vi "RT Main.vi"() -> ()   [LabVIEW 2021]
doc: "This example monitors the myRIO onboard button and increments or decrements the number below based on the Direction control."
uses:
  <vilib>/myRIO/Express VI/Onboard Devices/LED/LED Express VI.xnode
  <vilib>/myRIO/Instrument Drivers/Onboard IO/DIO/vis/Write.vi
  <vilib>/myRIO/Instrument Drivers/Onboard IO/DIO/DIO.lvlib
  <vilib>/myRIO/Common/Instrument Driver Framework/myRIO v1.0/DIO/typedefs/DIO Channels Enum.ctl
  <vilib>/myRIO/Common/Instrument Driver Framework/myRIO v1.0/DIO/typedefs/DIO Channels List.ctl
  <vilib>/myRIO/Common/Instrument Driver Framework/Utilities/typedefs/Generic FPGA Reference.ctl
  <vilib>/myRIO/Common/Instrument Driver Framework/Utilities/typedefs/myRIO v1.0 Reference.ctl
  <vilib>/myRIO/Common/Instrument Driver Framework/Utilities/typedefs/Hardware Version Enum.ctl
  <vilib>/myRIO/Common/Instrument Driver Framework/Utilities/typedefs/myRIO Generic Hardware Reference.ctl
  <vilib>/myRIO/Instrument Drivers/Onboard IO/DIO/typedefs/DIO Reference.ctl
  <vilib>/myRIO/Instrument Drivers/Onboard IO/DIO/vis/myRIO DIO Open.xnode
  <vilib>/myRIO/Common/Instrument Driver Framework/Utilities/vis/Is FPGA Ref Available.vi
  <vilib>/myRIO/Common/Instrument Driver Framework/myRIO v1.0/DIO/vis/myRIO v1.1 Open DIO.vi
  <vilib>/userdefined/High Color/nirio_resource_hc.ctl
panel:
  out "Axis Info":cluster{"X axis":i32, "Y axis":i32}[](graph)
  out "Pov Direction":picture
  out "Button 4":bool
  out "Button 3":bool
  out "Button 2":bool
  out "Button 1":bool
  in  "Device Index":i8
  out "error out":errorcluster
  in  "Stop":bool
  # "Overview: This VI demonstrates how to monitor the activity of the joystick connected to the myRIO.\nInstructions:\n1.\tIn the Project Explorer window, verify the IP address of the myRIO target. If it is incorrect, \nupdate the IP address.\n2. Connect a joystick to the myRIO through the USB port.\n3. Run the VI.\n4.\tPush the buttons and axes on the joystick and observe the indicators of the VI."
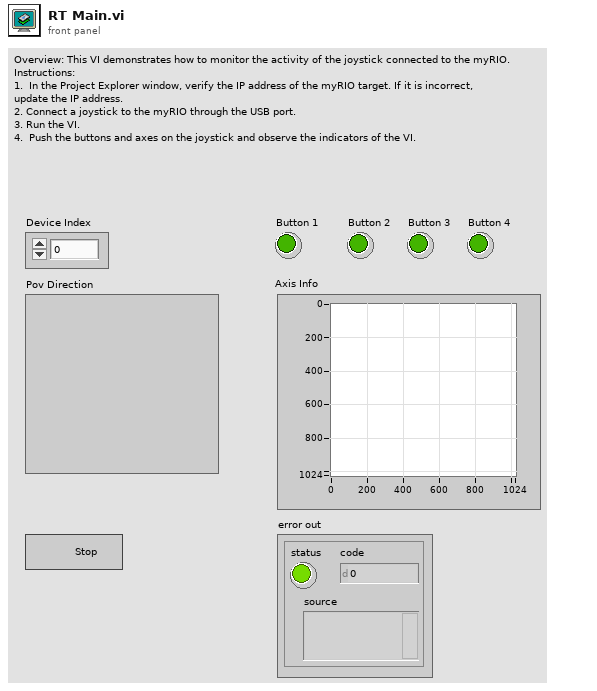
[diagram p1: front panel]
types:
  T1 = typedef "DIO.lvlib/DIO Reference.ctl" = cluster{"myRIO Reference":T2, "DIO Channels List":T6}
  T2 = typedef "myRIO Generic Hardware Reference.ctl" = cluster{"myRIO Model":T3, "myRIO Hardware Reference":T4}
  T3 = typedef "Hardware Version Enum.ctl" = enum16{"Unknown", "myRIO-1900", "myRIO-1950", "roboRIO", "NI ELVIS RIO CM", "ELVIS III"}
  T4 = typedef "myRIO v1.0 Reference.ctl" = cluster{"Generic FPGA Reference":T5, "Allow multiple opens":bool}
  T5 = typedef "Generic FPGA Reference.ctl" = refnum<k20>
  T6 = typedef "DIO Channels List.ctl" = T7[]
  T7 = typedef "DIO Channels Enum.ctl" = enum16{"Not Connected", "C/DIO0", "C/DIO1", "C/DIO2", "C/DIO3", "C/DIO4", "C/DIO5", "C/DIO6", "C/DIO7", "A/DIO0", "A/DIO1", "A/DIO2", "A/DIO3", "A/DIO4", "A/DIO5", "A/DIO6", "A/DIO7", "A/DIO8", "A/DIO9", "A/DIO10", "A/DIO11", "A/DIO12", "A/DIO13", "A/DIO14", "A/DIO15", "A/DIO16", "A/DIO17", "A/DIO18", "A/DIO19", "B/DIO0", "B/DIO1", "B/DIO2", "B/DIO3", "B/DIO4", "B/DIO5", "B/DIO6", "B/DIO7", "B/DIO8", "B/DIO9", "B/DIO10", "B/DIO11", "B/DIO12", "B/DIO13", "B/DIO14", "B/DIO15", "B/DIO16", "B/DIO17", "B/DIO18", "B/DIO19", "LED0", "LED1", "LED2", "LED3", "Button0", "DIO/DIO0", "DIO/DIO1", "DIO/DIO2", "DIO/DIO3", "DIO/DIO4", "DIO/DIO5", "DIO/DIO6", "DIO/DIO7", "DIO/DIO8", "DIO/DIO9", "SPI/CS0", "SPI/CS1", "SPI/CS2", "SPI/CS3", "LED RADIO (Green)", "LED RADIO (Red)", "LED COMM (Green)", "LED COMM (Red)", "LED MODE (Green)", "LED MODE (Red)"}
  T8 = typedef "nirio_resource_hc.ctl" = tag
  T9 = cluster{"X axis":i32, "Y axis":i32, "Z axis":i32, "X axis rotation":i32, "Y axis rotation":i32, "Z axis rotation":i32, "U axis":i32, "V axis":i32}
  T10 = cluster{"button 1":bool, "button 2":bool, "button 3":bool, "button 4":bool, "button 5":bool, "button 6":bool, "button 7":bool, "button 8":bool, "button 9":bool, "button 10":bool, "button 11":bool, "button 12":bool, "button 13":bool, "button 14":bool, "button 15":bool, "button 16":bool, "button 17":bool, "button 18":bool, "button 19":bool, "button 20":bool, "button 21":bool, "button 22":bool, "button 23":bool, "button 24":bool, "button 25":bool, "button 26":bool, "button 27":bool, "button 28":bool, "button 29":bool, "button 30":bool, "button 31":bool, "button 32":bool}
  T11 = cluster{"pov 1":i32, "pov 2":i32, "pov 3":i32, "pov 4":i32}
  T12 = typedef "LVBoundsTypeDef.ctl" = cluster{"Width":u32, "Height":u32}
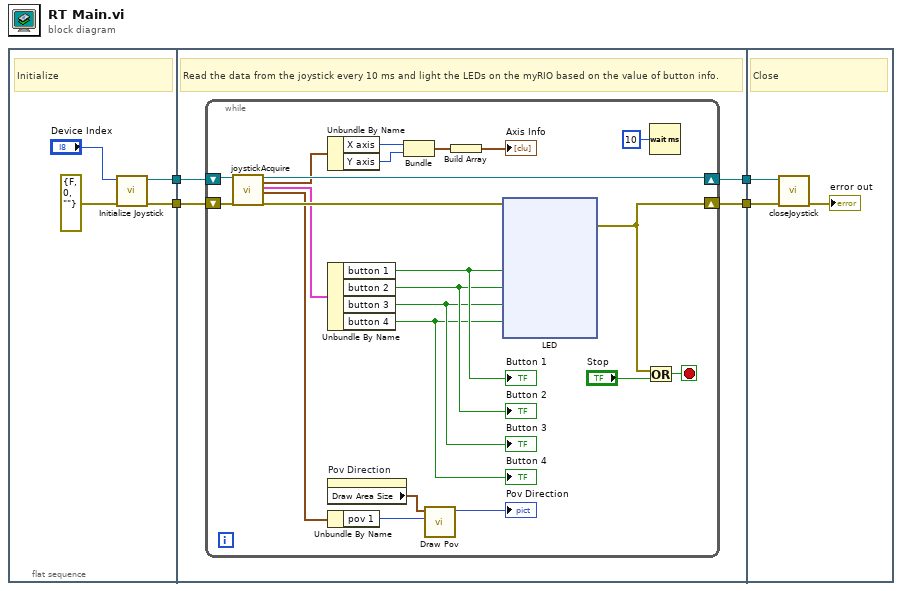
[diagram p0: block diagram]
diagram:
  n1 = flat-sequence {
    tunnel: [w7] -> w3
    tunnel: [w5] -> w2
    tunnel: [w12] -> w4
    tunnel: w3 -> [w11]
    tunnel: w2 -> [w10]
    tunnel: [w9] -> w1
    tunnel: w4 -> [w75]
    tunnel: w1 -> [w73]
    frame #0 {
      # "Initialize"
      n2 = call <vilib>:"Initialize Joystick.vi"("error in (no error)"=errorcluster {"status"=FALSE, "code"=0, "source"=""} ("error out"), "device index"="Device Index") -> ("error out"=w7:errorcluster, "device ID"=w5:refnum<k1>)  [unwired: 8 in]
    }
    frame #1 {
      # "Read the data from the joystick every 10 ms and light the LEDs on the myRIO based on the value of button info."
      n3 = while {
        shift-right: [w28] -> w12
        shift-left: w11 -> [w31]
        shift-right: [w26] -> w9
        shift-left: w10 -> [w30]
        stop <- w34 stop-if-true
        n4 = call <vilib>:"joystickAcquire.vi"("device ID"=w30, "error in (no error)"=w31) -> ("device ID"=w26:refnum<k1>, "axis info"=w25:T9, "button info"=w27:T10, "direction info"=w24:T11, "error out"=w29:errorcluster)  [unwired: 13 in]
        n5 = Unbundle By Name(w25) -> ("X axis"=w16:i32, "Y axis"=w15:i32)
        n6 = Unbundle By Name(w27) -> ("button 1"=w23:bool, "button 2"=w22:bool, "button 3"=w21:bool, "button 4"=w20:bool)
        "Button 1" <- w23
        "Button 2" <- w22
        "Button 3" <- w21
        "Button 4" <- w20
        n7 = property on="Pov Direction" class="Pict"() -> ("Draw Area Size"=w17:T12)  [unwired: 2 in, 2 out]
        n8 = Unbundle By Name(w24) -> ("pov 1"=w18:i32)
        n9 = Bundle("X axis"=w16, "Y axis"=w15) -> (w14:cluster{"X axis":i32, "Y axis":i32})  [unwired: 1 in]
        n10 = call "Draw Pov.vi"("pov"=w18, "Draw Area Size"=w17) -> ("2D Picture"=→"Pov Direction":picture)  [unwired: 9 in]
        n11 = Build Array(w14) -> (→"Axis Info":cluster{"X axis":i32, "Y axis":i32}[])
        n12 = xnode "LED"("LED0"=w23, "LED1"=w22, "LED2"=w21, "LED3"=w20, "error in (no error)"=w29) -> ("error out"=w28:errorcluster)
        n13 = Or(x=w28, y="Stop") -> (x .or. y?=w34:bool)
        n14 = Wait (ms)(milliseconds to wait=u32 10) -> ()  [unwired: 1 out]
      }
    }
    frame #2 {
      # "Close"
      n15 = call <vilib>:"closeJoystick.vi"("error in (no error)"=w75, "device ID"=w73) -> ("error out"=→"error out":errorcluster)  [unwired: 8 in]
    }
  }
